vi "Panel Resized.vi"(6 "Sizing Refnums":T2, 8 "error in (no error)":errorcluster, 9 "Origin":cluster{"H":i16, "V":i16}, 10 "NewBnds":T1, 11 "Size Constraints":cluster{"min tab width":i32, "w/h":dbl}) -> (0 "error out":errorcluster)   [LabVIEW 2016]
uses:
  <vilib>/Utility/miscctls.llb/LVRectTypeDef.ctl
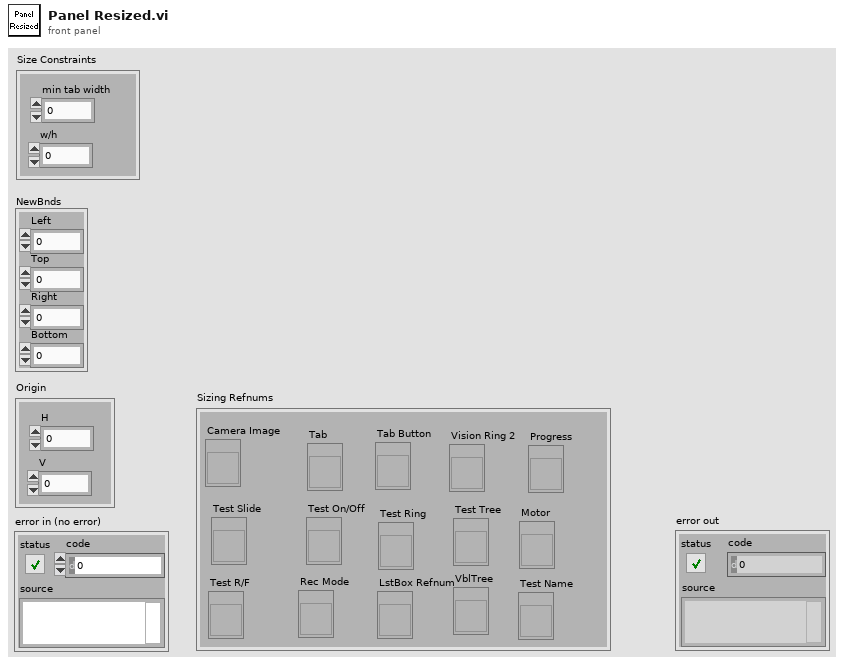
[diagram p1: front panel]
types:
  T1 = typedef "LVRectTypeDef.ctl" = cluster{"Left":i16, "Top":i16, "Right":i16, "Bottom":i16}
  T2 = cluster{"Camera Image":refnum<vi>, "Tab":refnum<vi>, "Tab Button":refnum<vi>, "Vision Ring 2":refnum<vi>, "Rec Mode":refnum<vi>, "Test Slide":refnum<vi>, "Test On/Off":refnum<vi>, "Test Ring":refnum<vi>, "Test R/F":refnum<vi>, "Test Name":refnum<vi>, "Motor":refnum<vi>, "Progress":refnum<vi>, "LstBox Refnum":refnum<vi>, "Test Tree":refnum<vi>, "VblTree":refnum<vi>}
  T3 = typedef "LVPositionTypeDef.ctl" = cluster{"Left":i32, "Top":i32}
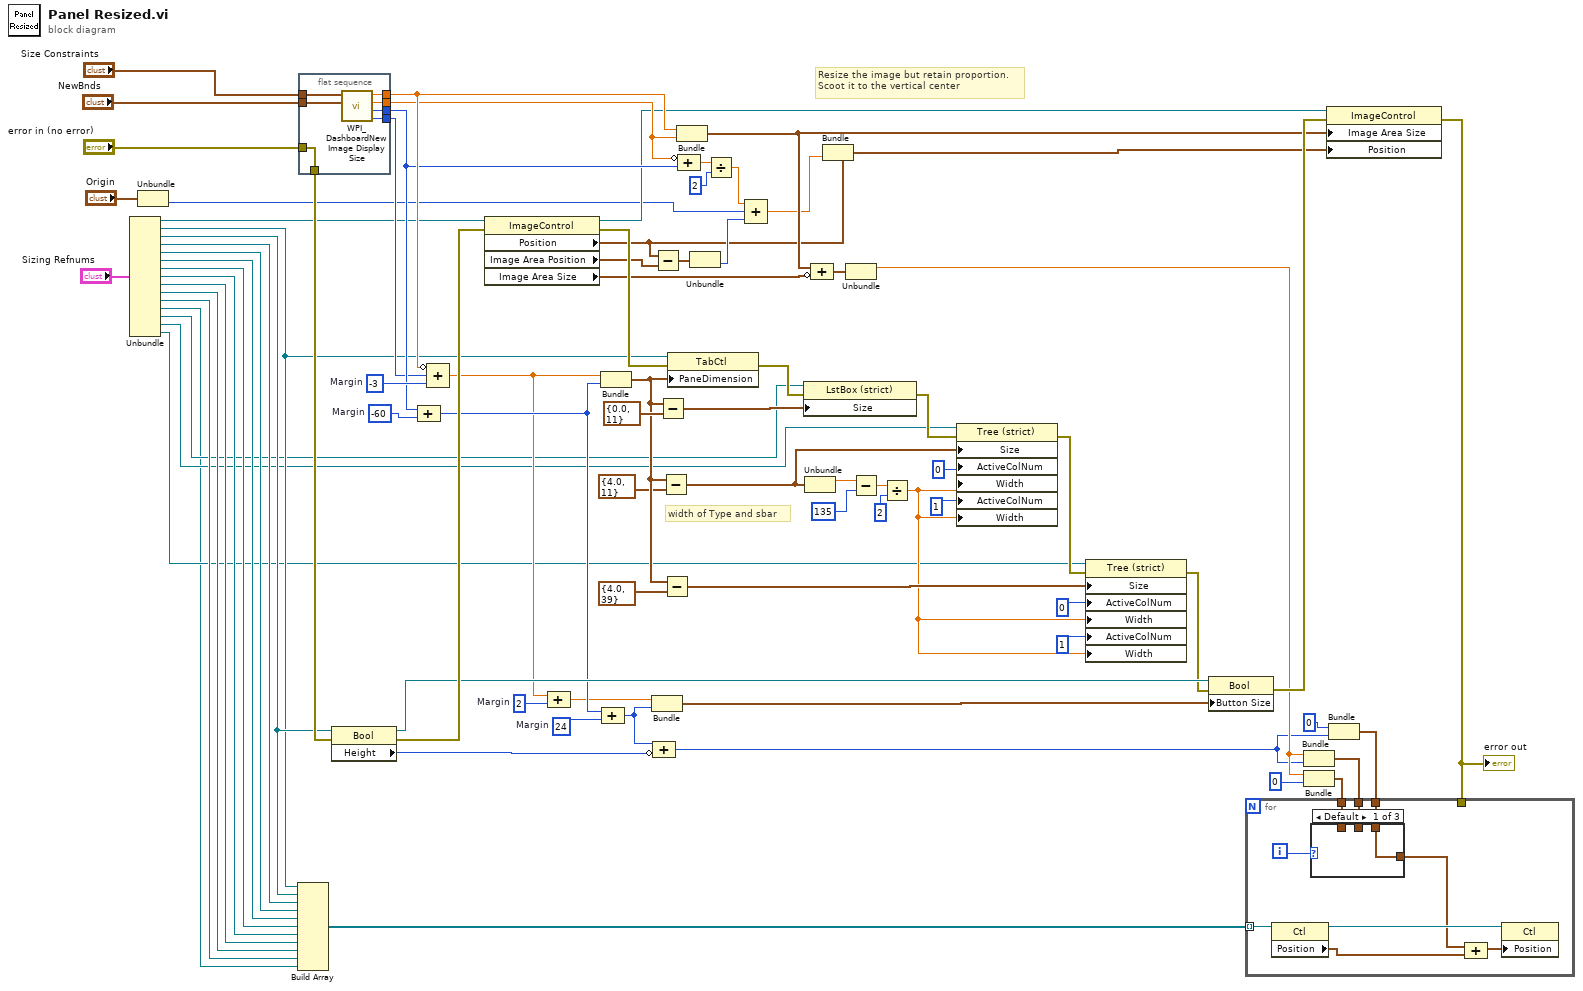
[diagram p0: block diagram]
diagram:
  w62 = 24  # Margin
  w60 = 2  # Margin
  w56 = -60  # Margin
  w66 = -3  # Margin
  # "width of Type and sbar"
  # "Resize the image but retain proportion.\nScoot it to the vertical center"
  n1 = Unbundle("Sizing Refnums") -> ("Camera Image"=w30:refnum<vi>, "Tab"=w31:refnum<vi>, "Tab Button"=w39:refnum<vi>, "Vision Ring 2"=w77:refnum<vi>, "Rec Mode"=w78:refnum<vi>, "Test Slide"=w79:refnum<vi>, "Test On/Off"=w80:refnum<vi>, "Test Ring"=w81:refnum<vi>, "Test R/F"=w82:refnum<vi>, "Test Name"=w9:refnum<vi>, "Motor"=w8:refnum<vi>, "Progress"=w1:refnum<vi>, "LstBox Refnum"=w2:refnum<vi>, "Test Tree"=w3:refnum<vi>, "VblTree"=w4:refnum<vi>)
  n2 = Unbundle("Origin") -> ("V"=w36:i16)  [unwired: 1 out]
  n3 = Build Array(w31, w39, w77, w78, w79, w80, w81, w82, w9, w8, w1) -> (w76:refnum<vi>[])
  n4 = flat-sequence {
    tunnel: "NewBnds" -> [w89]
    tunnel: "Size Constraints" -> [w88]
    tunnel: [w87] -> w55
    tunnel: [w86] -> w63
    tunnel: [w85] -> w64
    tunnel: [w84] -> w65
    tunnel: [w83] -> w75
    tunnel: "error in (no error)" -> [w83]
    frame #0 {
      n5 = call <vilib>:"WPI_DashboardNew Image Display Size.vi"("NewBnds"=w89, "Size Constraints"=w88) -> ("Window Width"=w87:i16, "Window Height"=w85:i16, "Height"=w86:dbl, "Width"=w84:dbl)  [unwired: 6 in]
    }
  }
  n6 = property class="Bool"(reference=w39, error in=w75) -> (reference out=w69:refnum<vi>, error out=w74:errorcluster, "Height"=w68:u32)
  n7 = Compound Arithmetic op=unknown(w64, w56) -> (w61:i32)
  n8 = Compound Arithmetic op=ADD(invert w65, w55, w66) -> (w59:dbl)
  n9 = property class="ImageControl"(reference=w30, error in=w74) -> (reference out=w48:refnum<vi>, error out=w72:errorcluster, "Position"=w47:T3, "Image Area Position"=w42:cluster{"Left":i32, "Top":i32}, "Image Area Size"=w53:cluster{"Width":u32, "Height":u32})
  n10 = Compound Arithmetic op=ADD(w59, w60) -> (w58:dbl)
  n11 = Bundle(w59, w61) -> (w26:cluster{dbl, i32})  [unwired: 1 in]
  n12 = Compound Arithmetic op=ADD(w61, w62) -> (w67:i32)
  n13 = Bundle(w58, w67) -> (w57:cluster{dbl, i32})  [unwired: 1 in]
  n14 = Subtract(x=w47, y=w42) -> (x-y=w49:T3)
  n15 = Compound Arithmetic op=ADD(w67, invert w68) -> (w7:u32)
  n16 = Subtract(x=w26, y=cluster{dbl, i32} {0.0, 11}) -> (x-y=w28:cluster{dbl, i32})
  n17 = Subtract(x=w26, y=cluster{dbl, i32} {4.0, 11}) -> (x-y=w17:cluster{dbl, i32})
  n18 = Subtract(x=w26, y=cluster{dbl, i32} {4.0, 39}) -> (x-y=w23:cluster{dbl, i32})
  n19 = property class="TabCtl"(reference=w31, error in=w72, "PaneDimension"=w26) -> (error out=w29:errorcluster)  [unwired: 1 out]
  n20 = Bundle("Width"=w65, "Height"=w63) -> (w51:cluster{"Width":dbl, "Height":dbl})  [unwired: 1 in]
  n21 = Compound Arithmetic op=ADD(invert w63, w64) -> (w43:dbl)
  n22 = Unbundle(w49) -> ("Top"=w50:i32)  [unwired: 1 out]
  n23 = Divide(x=w43, y=2) -> (x/y=w45:dbl)
  n24 = Compound Arithmetic op=ADD(w45, w36, w50) -> (w46:dbl)
  n25 = property class="LstBox (strict)"(reference=w2, error in=w29, "Size"=w28) -> (error out=w22:errorcluster)  [unwired: 1 out]
  n26 = Unbundle(w17) -> (w16:dbl)  [unwired: 1 out]
  n27 = Compound Arithmetic op=ADD(w51, invert w53) -> (w54:cluster{"Width":dbl, "Height":dbl})
  n28 = Bundle(cluster=w47, "Top"=w46) -> (w52:T3)  [unwired: 1 in]
  n29 = Unbundle(w54) -> ("Width"=w70:dbl)  [unwired: 1 out]
  n30 = Subtract(x=w16, y=135 ("Active Cell:Active Column Number")) -> (x-y=w12:dbl)
  n31 = Divide(x=w12, y=2 ("Active Cell:Active Column Number")) -> (x/y=w10:dbl)
  n32 = property class="Tree (strict)"(reference=w3, error in=w22, "Size"=w17, "ActiveColNum"=0 ("Active Cell:Active Column Number"), "Width"=w10, "ActiveColNum"=1 ("Active Cell:Active Column Number"), "Width"=w10) -> (error out=w21:errorcluster)  [unwired: 1 out]
  n33 = property class="Tree (strict)"(reference=w4, error in=w21, "Size"=w23, "ActiveColNum"=0 ("Active Cell:Active Column Number"), "Width"=w10, "ActiveColNum"=1 ("Active Cell:Active Column Number"), "Width"=w10) -> (error out=w20:errorcluster)  [unwired: 1 out]
  n34 = property class="Bool"(reference=w69, error in=w20, "Button Size"=w57) -> (error out=w73:errorcluster)  [unwired: 1 out]
  n35 = Bundle("Width"=w70, w7) -> (w41:cluster{"Width":dbl, u32})  [unwired: 1 in]
  n36 = Bundle("Width"=w70, 0) -> (w40:cluster{"Width":dbl, i32})  [unwired: 1 in]
  n37 = property class="ImageControl"(reference=w48, error in=w73, "Image Area Size"=w51, "Position"=w52) -> (error out=w35:errorcluster)  [unwired: 1 out]
  "error out" <- w35
  n38 = Bundle(0, w7) -> (w5:cluster{i32, u32})  [unwired: 1 in]
  n39 = for {
    tunnel: w76 -> [w98] mode=indexing
    tunnel: w41 -> [w92]
    tunnel: w40 -> [w93]
    tunnel: w35 -> [_]
    tunnel: w5 -> [w91]
    i -> [w94]
    n40 = property class="Ctl"(reference=w98) -> (reference out=w97:refnum<vi>, "Position"=w96:T3)  [unwired: 1 in, 1 out]
    n41 = case shown="Default" w94 {
      tunnel: w93 -> [_ w100 _]
      tunnel: w92 -> [_ _ w101]
      tunnel: w91 -> [w99 _ _]
      tunnel: [w99 w100 w101] -> w90
      frame Default {
      }
      frame 0, 1 {
      }
      frame 2, 3 {
      }
    }
    n42 = Compound Arithmetic op=ADD(w90, w96) -> (w95:cluster{dbl, u32})
    n43 = property class="Ctl"(reference=w97, "Position"=w95) -> ()  [unwired: 1 in, 2 out]
  }
